vi "Set Measurement Configuration.vi"(8 "error in (no error)":errorcluster, 10 "Measurement Configuration":T1={"Function"=enum."2-Wire Resistance", " Manual Resolution"=enum."6.5", "Frequency Source"=enum."AC Voltage", "Auto Range"=enum."ON"}, 11 "Agilent 3458A in":refnum<class "Agilent 3458A.lvclass">) -> (0 "error out":errorcluster, 3 "Agilent 3458A out":refnum<class "Agilent 3458A.lvclass">)   [LabVIEW 2011, in "Agilent 3458A.lvclass"]
uses:
  Agilent 3458A.lvclass
  Measurement Configuration.ctl
  <instrlib>/Agilent 3458/Agilent 3458.lvlib
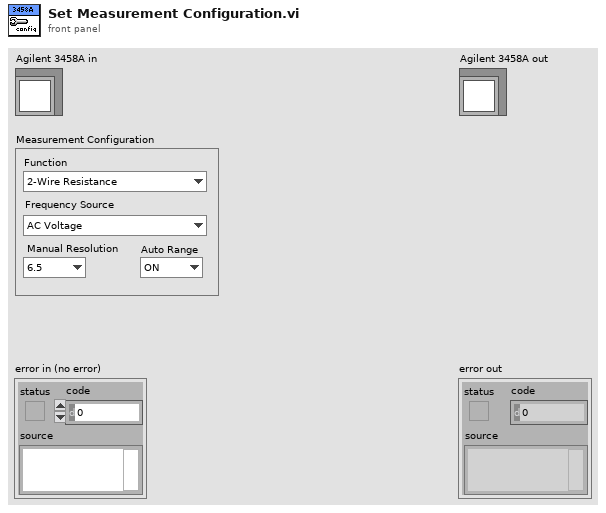
[diagram p1: front panel]
types:
  T1 = typedef "Agilent 3458A.lvclass/Measurement Configuration.ctl" = cluster{"Function":enum16{"DC Voltage", "AC Voltage", "AC + DC Voltage", "DC Current", "AC Current", "AC + DC Current", "2-Wire Resistance", "4-Wire Resistance", "Frequency", "Period", "Direct Sampling DC", "Direct Sampling AC", "Sub-Sampling DC", "Sub-Sampling AC"}, " Manual Resolution":enum16{"4.5", "5.5", "6.5", "7.5", "8.5"}, "Frequency Source":enum16{"AC + DC Current", "AC + DC Voltage", "AC Current", "AC Voltage"}, "Auto Range":enum16{"OFF", "ON", "ONCE"}}
  T2 = enum16{"DC Voltage", "AC Voltage", "AC + DC Voltage", "DC Current", "AC Current", "AC + DC Current", "2-Wire Resistance", "4-Wire Resistance", "Frequency", "Period", "Direct Sampling DC", "Direct Sampling AC", "Sub-Sampling DC", "Sub-Sampling AC"}
  T3 = enum16{"AC + DC Current", "AC + DC Voltage", "AC Current", "AC Voltage"}
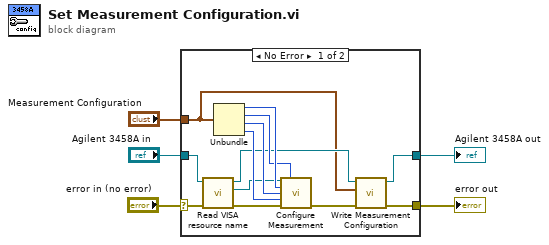
[diagram p0: block diagram]
diagram:
  n1 = case shown="No Error" "error in (no error)" {
    selector: "error in (no error)" -> [w13 w20]
    tunnel: [w9 w20] -> w4
    tunnel: [w6 w19] -> w2
    tunnel: "Agilent 3458A in" -> [w14 w19]
    tunnel: "Measurement Configuration" -> [w7 _]
    frame No Error {
      n2 = call-dynamic "Read VISA resource name.vi"("error in (no error)"=w13, "Multimeter in"=w14) -> ("error out"=w12:errorcluster, "VISA resource name"=w11:refnum<visa-resource-name>, "Multimeter out"=w8:refnum<class "Agilent 3458A.lvclass">)  [unwired: 7 in]
      n3 = Unbundle(w7) -> ("Function"=w18:T2, "Manual Resolution"=w17:enum16{"4.5", "5.5", "6.5", "7.5", "8.5"}, "Frequency Source"=w16:T3, "Auto Range"=w15:enum16{"OFF", "ON", "ONCE"})
      n4 = call <instrlib>:"Configure Measurement.vi"("VISA resource name"=w11, "Manual Resolution (2: 6.5 digits)"=w17, "Function (0: DC Voltage)"=w18, "Frequency Source (3: AC Voltage)"=w16, "Auto Range (1:ON)"=w15, "error in (no error)"=w12) -> ("error out"=w10:errorcluster)  [unwired: 8 in, 1 out]
      n5 = call-dynamic "Write Measurement Configuration.vi"("error in (no error)"=w10, "Measurement Configuration"=w7, "Agilent 3458A in"=w8) -> ("error out"=w9:errorcluster, "Agilent 3458A out"=w6:refnum<class "Agilent 3458A.lvclass">)  [unwired: 7 in]
    }
    frame Error {
    }
  }
  "error out" <- w4
  "Agilent 3458A out" <- w2
